vi "IPS Set Activity.vi"(4 "Error In":errorcluster, 6 "Set Activity":T1, 7 "VISA resource name":refnum<visa-resource-name>="GPIB1::25::INSTR") -> (0 "Error Out":errorcluster, 2 "Response":string="A\r", 3 "VISA resource name":refnum<visa-resource-name>="GPIB1::25::INSTR")   [LabVIEW 2016, in "IPS-120.lvlib"]
uses:
  IPS-120.lvlib
  Typedefs/Set Activity - Enum.ctl
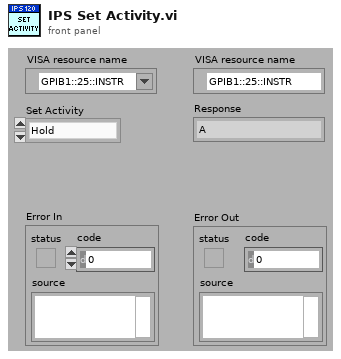
[diagram p1: front panel]
types:
  T1 = typedef "IPS-120.lvlib/Set Activity - Enum.ctl" = enum16{"Hold", "To Set Point", "To Zero", "Clamp"}
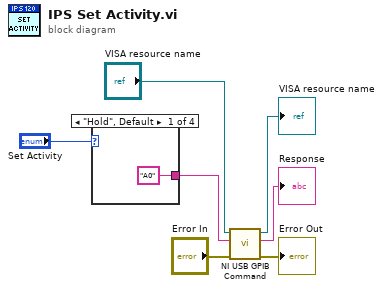
[diagram p0: block diagram]
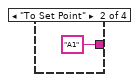
[diagram p2: hidden frame]
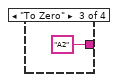
[diagram p3: hidden frame]
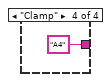
[diagram p4: hidden frame]
diagram:
  n1 = case shown="\"Hold\", Default" "Set Activity" {
    tunnel: ["A0" "A1" "A2" "A4"] -> w4
    frame "Hold", Default {
    }
    frame "To Set Point" {
    }
    frame "To Zero" {
    }
    frame "Clamp" {
    }
  }
  n2 = call "NI USB GPIB Command.vi"("Error In"="Error In", "write buffer"=w4, "VISA resource name"="VISA resource name") -> ("Error Out"=→"Error Out":errorcluster, "read buffer"=→"Response":string, "VISA resource name out"=→"VISA resource name":refnum<visa-resource-name>)  [unwired: 6 in]
